vi "Actor Core.vi"(8 "error in":errorcluster, 11 "CharmView in":refnum<class "CharmView.lvclass">) -> (0 "error out":errorcluster, 3 "Actor out":refnum<class "Actor.lvclass">)   [LabVIEW 2012, in "Win8uiFramework.lvlib" / "CharmView.lvclass"]
doc: "(<B>Filename</B>: Actor Framework.lvlib:Actor.lvclass:Actor Core.vi)\n\nReceives messages to the actor, reacts to them, and initiates any error handling that may shut the actor down.\n\nDescendant classes may override this VI to append parallel tasks for the actor to complete while it handles messages. Overrides use the Call Parent Method node."
uses:
  CharmView.lvclass
  <vilib>/ActorFramework/Actor/Actor.lvclass
  ViewableActor.lvclass
panel:
  out "Time":string="Settings"
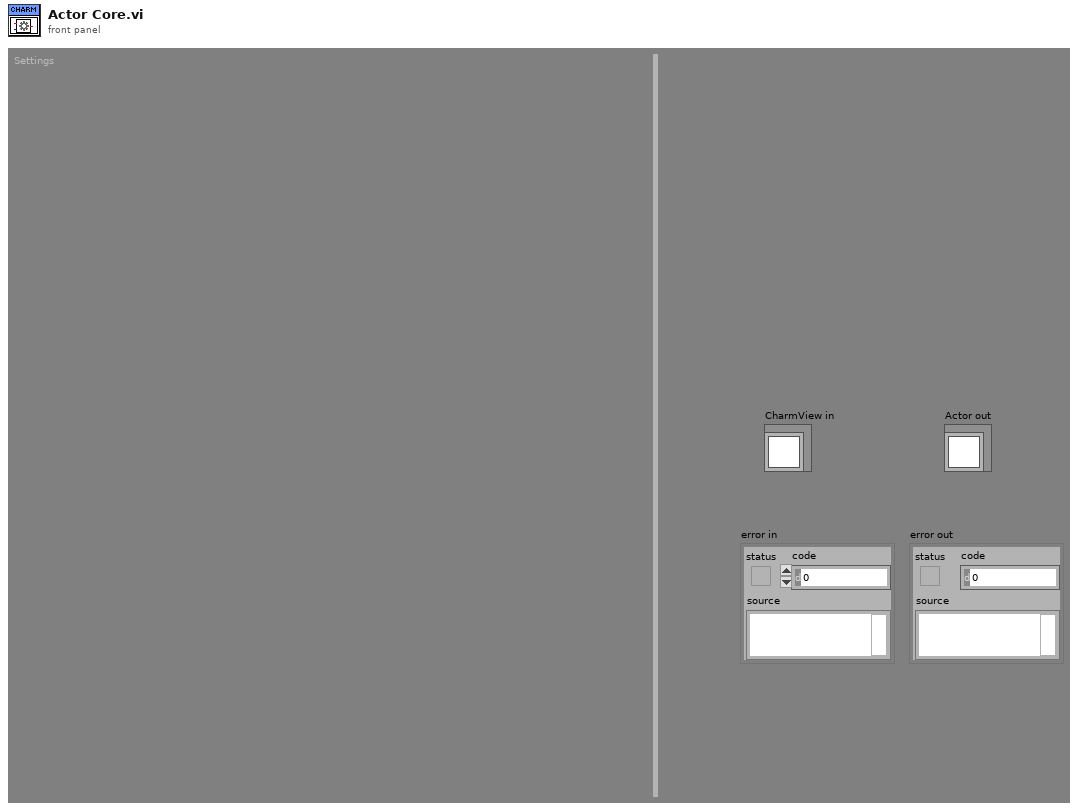
[diagram p1: front panel]
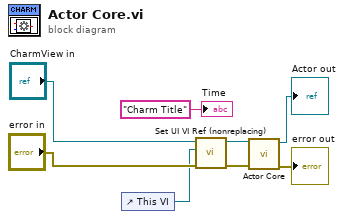
[diagram p0: block diagram]
diagram:
  n1 = control-ref of="This VI"() -> (w2:refnum<vi>)
  n2 = call "Set UI VI Ref (nonreplacing).vi"("error in (no error)"="error in", "UI VI Ref"=w2, "ViewableActor in"="CharmView in") -> ("error out"=w1:errorcluster, "ViewableActor out"=w5:refnum<class "CharmView.lvclass">)  [unwired: 6 in, 1 out]
  n3 = call-parent "Actor Core.vi"("error in"=w1, "Actor in"=w5) -> ("error out"=→"error out":errorcluster, "Actor out"=→"Actor out":refnum<class "Actor.lvclass">)  [unwired: 8 in]
  "Time" <- "Charm Title" ("Time")
